vi "Get CustomDevice Reference.vi"(8 "error in":errorcluster, 11 "Node Ptr":T1 format="%.0x") -> (0 "error out":errorcluster, 2 "Custom Device":refnum<k24>, 3 "Node Ptr":T1 format="%.0x")   [LabVIEW 2026]
uses:
  <vilib>/NI VeriStand/Custom Device API/Custom Device Item Ref.ctl
  NationalInstruments.VeriStand.SystemDefinitionAPI
  <vilib>/NI VeriStand/Custom Device API/Custom Device API.lvlib
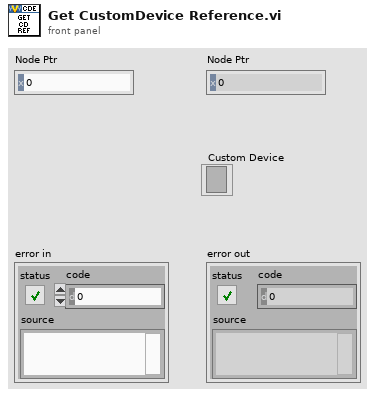
[diagram p1: front panel]
types:
  T1 = typedef "Custom Device API.lvlib/Custom Device Item Ref.ctl" = u64
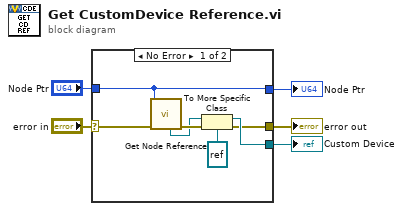
[diagram p0: block diagram]
diagram:
  n1 = case shown="No Error" "error in" {
    selector: "error in" -> [w7 w14]
    tunnel: [w6 w14] -> w4
    tunnel: "Node Ptr" -> [w12 w13]
    tunnel: [w12 w13] -> w2
    tunnel: [w8 _] -> w1
    frame No Error {
      n2 = call "Get Node Reference.vi"("error in"=w7, "Node Ptr"=w12) -> ("error out"=w11:errorcluster, "Base Node"=w10:refnum<k24>)  [unwired: 6 in, 2 out]
      n3 = To More Specific Class(target class=refnum<k24> refnum ("IDToCustomDevice"), reference=w10, error in=w11) -> (specific class reference=w8:refnum<k24>, error out=w6:errorcluster)
    }
    frame Error {
    }
  }
  "error out" <- w4
  "Node Ptr" <- w2
  "Custom Device" <- w1
